vi "rotation_to_axis_perm.vi"(11 "Rotation matrix (T)":T1 format="%#.3f") -> (1 "Residue matrix (R)":T1 format="%#.3f", 2 "Permutation vector":i32[](array[numeric])=[0, -16, 4], 3 "Permutation matrix (P)":T1 format="%#.3f")   [LabVIEW 2013]
uses:
  <vilib>/Analysis/Matrix/Datatypes/RealMatrix.ctl
  <vilib>/Analysis/baseanly.llb/Real A x B.vi
  <vilib>/Analysis/Matrix/Numeric/Conversions/Array To Matrix - RA2.vi
  <vilib>/Analysis/Matrix/NI_Matrix.lvlib
  <vilib>/Analysis/NI_AALBase.lvlib
  <vilib>/Analysis/Matrix/Numeric/Subtract/Subtract - RM,RM.vi
panel:
  out "Check":T1 format="%#_3g"
  # "Permutation vector represents the effect of the permutation, expressing, for each output axis, the corresponding input axis.  Indexing is one-based so that sign can encode whether there is a sign flip."
  # "Factor a rotation matrix T so that:\n   T = P * R\n\nWhere P permutes and/or sign flips axes (equivalent to 90 degree rotations and perhaps reflection).   This is a useful way to factor matrices which are nearly some combination of 90 degree rotations, as it results in a residue with all small angles, which is easier to interperet, for example as Euler angles."
  # "If result is correct, this will be all zeros.  Enable in diagram to check."
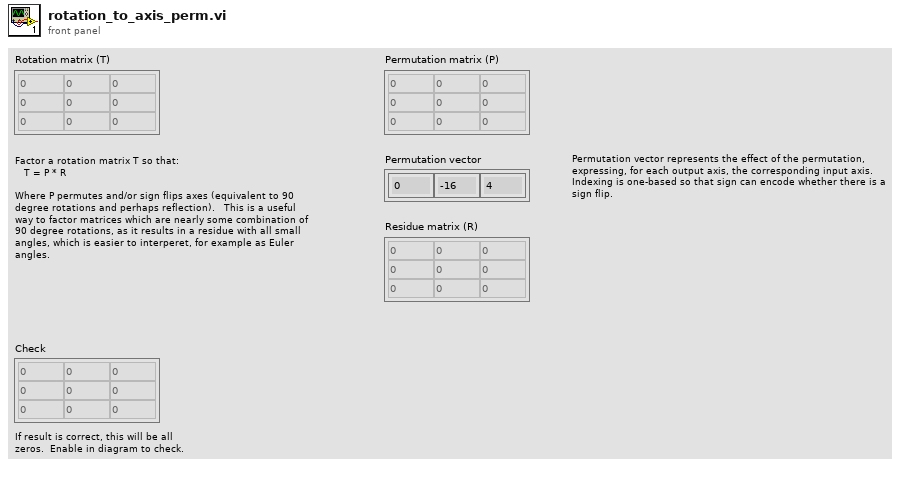
[diagram p1: front panel]
types:
  T1 = typedef "NI_Matrix.lvlib/RealMatrix.ctl" = dbl[][]
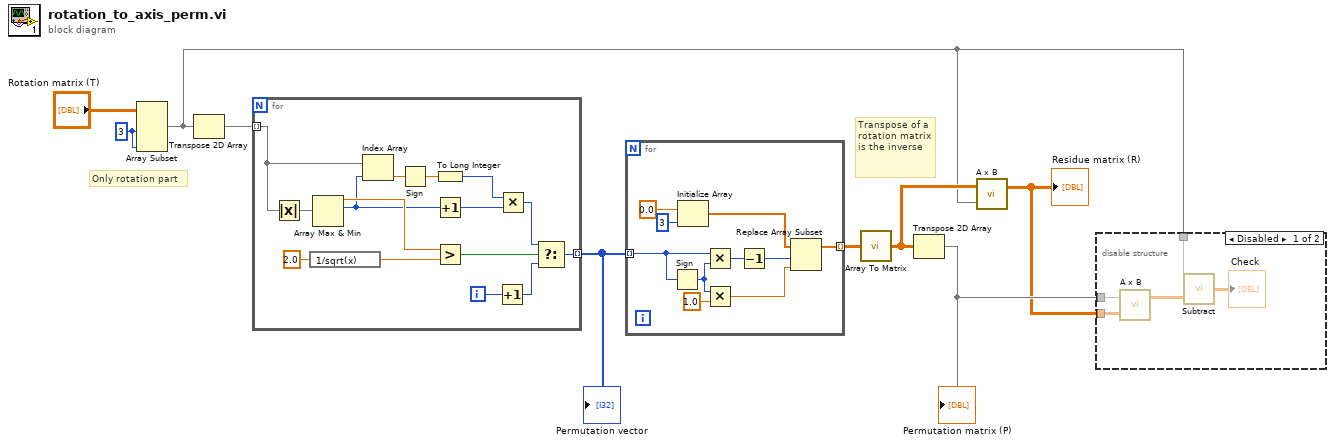
[diagram p0: block diagram]
diagram:
  w6 = 3 ("length")
  # "Transpose of a rotation matrix is the inverse"
  # "Only rotation part"
  n1 = Array Subset(array="Rotation matrix (T)", length (row)=w6, length (col)=w6) -> (w1:T1)  [unwired: 2 in]
  n2 = Transpose 2D Array(2D array=w1) -> (transposed array=w9:T1)
  n3 = for {
    tunnel: w9 -> [w23] mode=indexing
    tunnel: [w16] -> w8 mode=indexing
    i -> [w13]
    n4 = Absolute Value(x=w23) -> (abs(x)=w24:dbl[])
    n5 = expression code="1/sqrt(x)"(2.0 ("x")) -> (w21:dbl)
    n6 = Array Max & Min(array=w24) -> (max value=w22:dbl, max index (indices)=w12:i32)  [unwired: 2 out]
    n7 = Index Array(array=w23, index=w12) -> (element=w20:dbl)
    n8 = Sign(1:w20) -> (0:w18:dbl)
    n9 = To Long Integer(number=w18) -> (32bit integer=w17:i32)
    n10 = Increment(x=w12) -> (x+1=w11:i32)
    n11 = Greater?(x=w22, y=w21) -> (0:w19:bool)
    n12 = Increment(x=w13) -> (x+1=w14:i32)
    n13 = Multiply(x=w17, y=w11) -> (x*y=w10:i32)
    n14 = Select(t=w10, s=w19, f=w14) -> (s? t:f=w16:i32)
  }
  "Permutation vector" <- w8
  n15 = for {
    tunnel: w8 -> [w31] mode=indexing
    tunnel: [w27] -> w5 mode=indexing
    n16 = Sign(1:w31) -> (0:w30:i32)
    n17 = Initialize Array(0.0 ("element"), 3 ("dimension size")) -> (w32:dbl[])
    n18 = Multiply(x=w31, y=w30) -> (x*y=w26:i32)
    n19 = Multiply(x=w30, y=1.0) -> (x*y=w28:dbl)
    n20 = Decrement(x=w26) -> (x-1=w25:i32)
    n21 = Replace Array Subset(array=w32, new element=w28, index=w25) -> (w27:dbl[])
  }
  n22 = call-poly <vilib>:"Array To Matrix.vi"("Real 2D Array"=w5) -> ("Real Matrix"=w2:T1)
  n23 = Transpose 2D Array(2D array=w2) -> (transposed array=w4:T1)
  "Permutation matrix (P)" <- w4
  n24 = call-poly <vilib>:"A x B.vi"("B"=w1, "A"=w2) -> ("A x B"=w3:T1)  [unwired: 1 out]
  "Residue matrix (R)" <- w3
  n25 = disable-structure shown="Disabled" {
    disable-tunnel: w4 -> [w39 _]
    disable-tunnel: w3 -> [w38 _]
    disable-tunnel: w1 -> [w35 _]
    frame Disabled {
      n26 = call-poly <vilib>:"A x B.vi"("B"=w38, "A"=w39) -> ("A x B"=w37:T1)  [unwired: 1 out]
      n27 = call-poly <vilib>:"Subtract.vi"("Real Matrix B"=w37, "Real Matrix A"=w35) -> ("A - B"=→"Check":T1)
    }
    frame Enabled {
    }
  }
